vi "Untitled 1.vi"() -> ()   [LabVIEW 2014]
panel:
  in  "stop":bool
  out "loop 2":i32
  out "loop1":i32
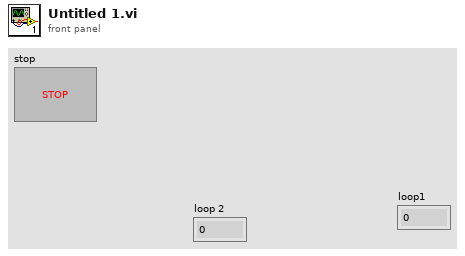
[diagram p1: front panel]
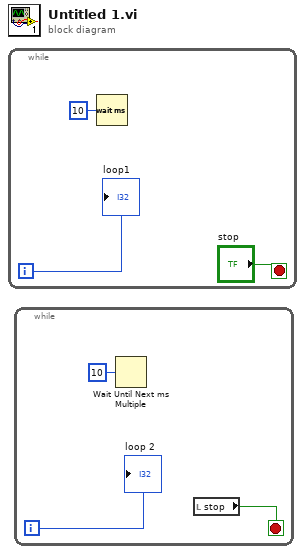
[diagram p0: block diagram]
diagram:
  n1 = while {
    i -> [w3]
    stop <- "stop" stop-if-true
    n2 = Wait (ms)(milliseconds to wait=u32 10) -> ()  [unwired: 1 out]
    "loop1" <- w3
  }
  n3 = while {
    i -> [w6]
    stop <- w5 stop-if-true
    n4 = Wait Until Next ms Multiple(millisecond multiple=u32 10) -> ()  [unwired: 1 out]
    n5 = local read "stop"() -> (w5:bool)
    "loop 2" <- w6
  }
